vi "Configure Sweep (Random).vi"(0 "VISA resource name":refnum<visa-resource-name>, 5 "Start Address (0)":u16 max=7999 step=1, 9 "Stop Address (0)":u16 max=7999 step=1, 11 "error in (no error)":errorcluster) -> (4 "VISA resource name out":refnum<visa-resource-name>, 15 "error out":errorcluster)   [LabVIEW 2017, in "ADCMT 6240.lvlib"]
doc: "This VI configures random memory sweep."
uses:
  ADCMT 6240.lvlib
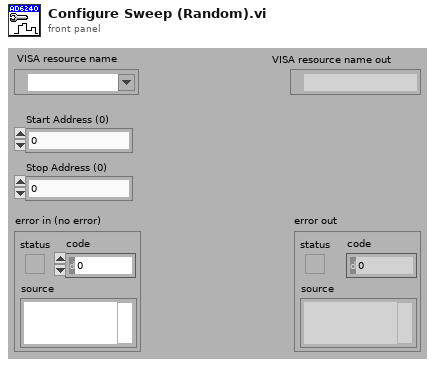
[diagram p1: front panel]
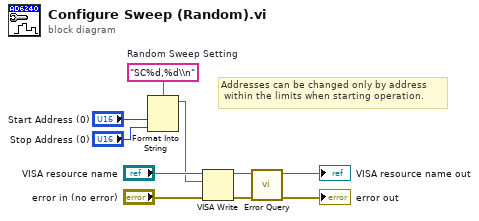
[diagram p0: block diagram]
diagram:
  w7 = "SC%d,%d\\n"  # Random Sweep Setting
  # "Addresses can be changed only by address\n within the limits when starting operation."
  n1 = Format Into String(format string=w7, "Start Address (0)", "Stop Address (0)") -> (resulting string=w1:string)  [unwired: 2 in, 1 out]
  n2 = VISA Write(VISA resource name="VISA resource name", write buffer=w1, error in (no error)="error in (no error)") -> (VISA resource name out=w5:refnum<visa-resource-name>, error out=w6:errorcluster)  [unwired: 1 out]
  n3 = call "Error Query.vi"("error in (no error)"=w6, "VISA resource name"=w5) -> ("error out"=→"error out":errorcluster, "VISA resource name out"=→"VISA resource name out":refnum<visa-resource-name>)  [unwired: 6 in, 2 out]
